vi "SP Set CH Reference.vi"(6 "Channel":i8=1 min=1 max=99 step=1, 8 "error in (no error)":errorcluster, 9 "CH Controls":T1={"Trace On"=TRUE, "Measure"=0, "Format"=0, "Autoscale"=TRUE, "Reference"=0.0, "\nRefUnit"="dB/Div", "Position"=5.0, "Scale"=10.0, "ScaleUnit"="dB/Div", "LimitOn"=TRUE, "LimitFill"=FALSE, "Display Data"=0, "Show Markers"=TRUE, "SXX"=""} {"Reference" format="%#.2g"; "Display Data" items=["Data", "Memory", "Data/Memory"]; "Format" items=["Log Mag", "Phase", "Expanded Phase", "Delay", "Smith", "Polar", "Lin Mag", "SWR", "Loss", "Real", "Imaginary"]; "Scale" min=0.001 step=1.0 format="%#.2g"; "Position" min=0.0 max=10.0}, 11 "Plot Reference":refnum<vi>) -> (0 "error out":errorcluster, 1 "dup CH Controls":T1={"Trace On"=TRUE, "Measure"=0, "Format"=0, "Autoscale"=TRUE, "Reference"=0.0, "\nRefUnit"="dB/Div", "Position"=5.0, "Scale"=10.0, "ScaleUnit"="dB/Div", "LimitOn"=TRUE, "LimitFill"=FALSE, "Display Data"=0, "Show Markers"=TRUE, "SXX"=""} {"Reference" format="%#.2g"; "Display Data" items=["Data", "Memory", "Data/Memory"]; "Format" items=["Log Mag", "Phase", "Expanded Phase", "Delay", "Smith", "Polar", "Lin Mag", "SWR", "Loss", "Real", "Imaginary"]; "Scale" min=0.001 step=1.0 format="%#.2g"; "Position" min=0.0 max=10.0}, 3 "dup Plot Reference":refnum<vi>)   [LabVIEW 2011]
uses:
  TypeDefs/SP Display Trace Controls.ctl
  TypeDefs/SP Display Format.ctl
  TypeDefs/SP Display Data.ctl
  TypeDefs/SP Plot Cluster Object.ctl
panel:
  # "Div"
  # "Div"
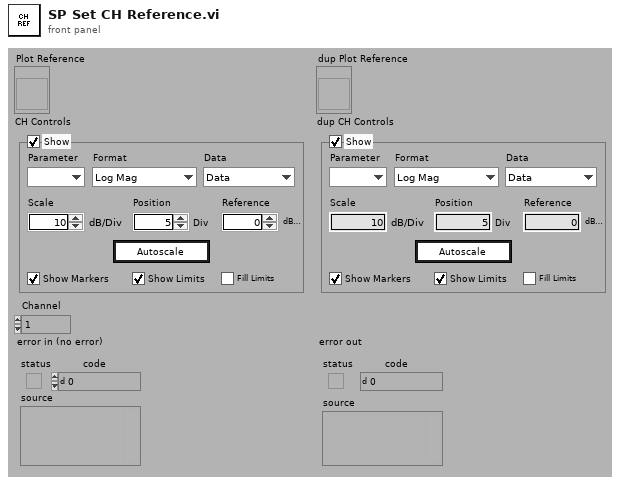
[diagram p1: front panel]
types:
  T1 = typedef "SP Display Trace Controls.ctl" = cluster{"Trace On":bool, "Measure":i32, "Format":T2, "Autoscale":bool, "Reference":dbl, "\nRefUnit":string, "Position":dbl, "Scale":dbl, "ScaleUnit":string, "LimitOn":bool, "LimitFill":bool, "Display Data":T3, "Show Markers":bool, "SXX":string}
  T2 = typedef "SP Display Format.ctl" = i32
  T3 = typedef "SP Display Data.ctl" = u16
  T4 = typedef "SP Plot Cluster Object.ctl" = enum16{"Plot", "CH Reference", "CH Label", "Start Label", "Stop Label", "Units Label", "Selected?", "CH Markers"}
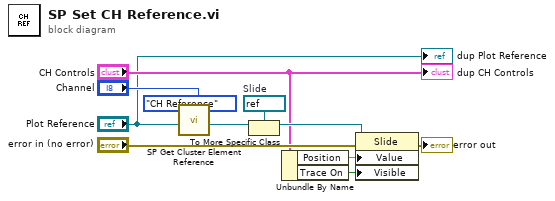
[diagram p0: block diagram]
diagram:
  w9 = refnum<vi> refnum  # Slide
  n1 = call "SP Get Cluster Element Reference.vi"("Channel"="Channel", "Element"=SP_Plot_Cluster_Object."CH Reference", "Plot Reference"="Plot Reference") -> ("Element Reference"=w8:refnum<vi>)  [unwired: 6 out]
  n2 = To More Specific Class(target class=w9, reference=w8) -> (specific class reference=w7:refnum<vi>)  [unwired: 1 in, 1 out]
  n3 = Unbundle By Name("CH Controls") -> ("Position"=w5:dbl, "Trace On"=w4:bool)
  n4 = property class="Slide"(reference=w7, error in="error in (no error)", "Value"=w5, "Visible"=w4) -> (error out=→"error out":errorcluster)  [unwired: 1 out]
  "dup CH Controls" <- "CH Controls"
  "dup Plot Reference" <- "Plot Reference"
